vi "gantry移動定位_六邊形(外切圓).vi"() -> ()   [LabVIEW 2016]
uses:
  Classes/Controller/Motion/A3200 Folder/A3200.lvclass
panel:
  out "點座標":dbl[][](array[numeric])
  in  "外切圓半徑":dbl=100.0
  in  "中心點座標":dbl[](array[numeric])
  out "Final Position":dbl[](array[numeric])
  out "Initial position":dbl[](array[numeric])
  in  "Speed (mm/s)":dbl=40.0
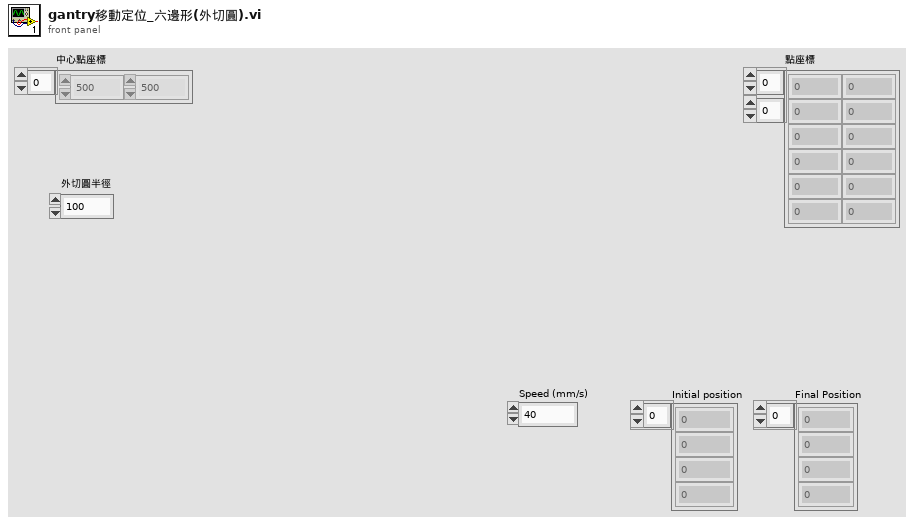
[diagram p1: front panel]
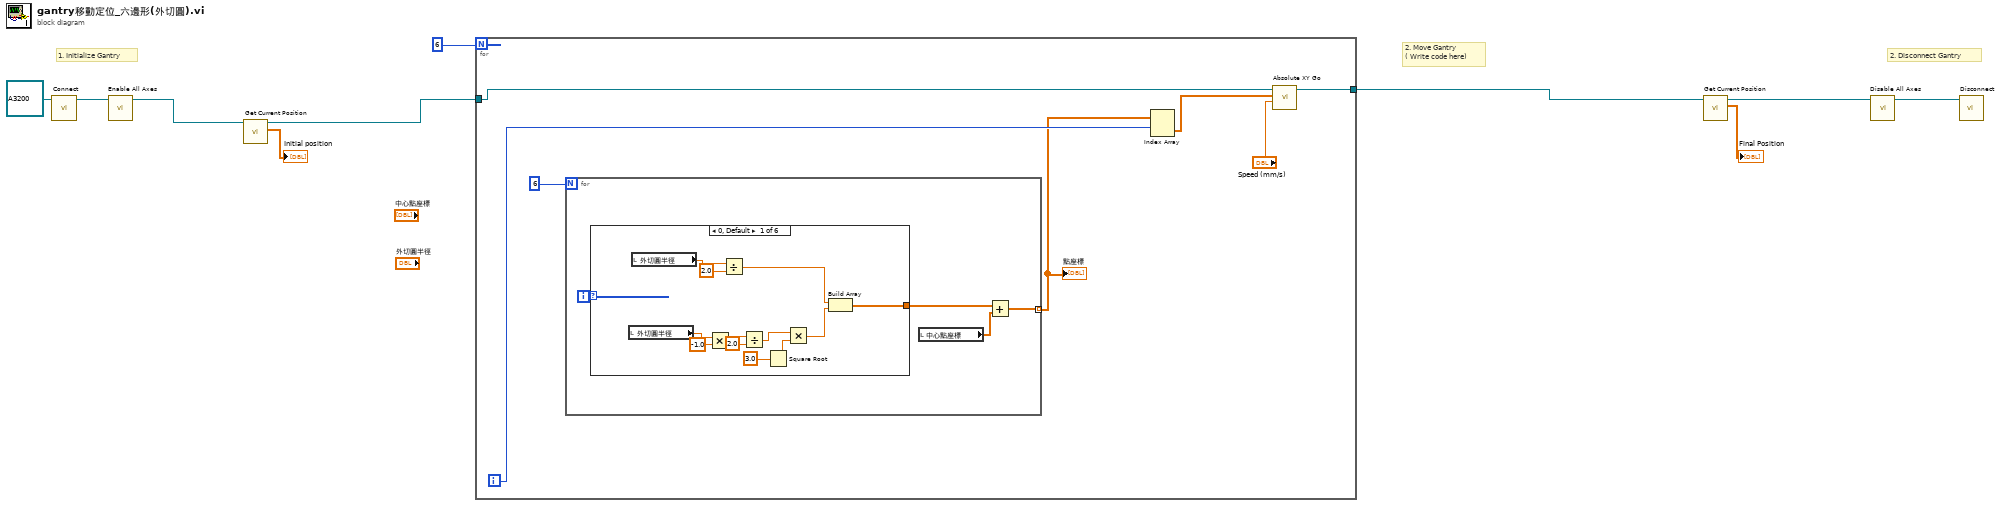
[diagram p0: block diagram]
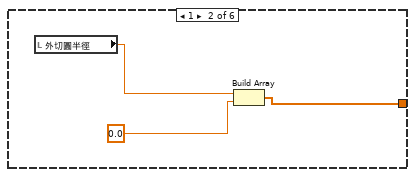
[diagram p2: hidden frame]
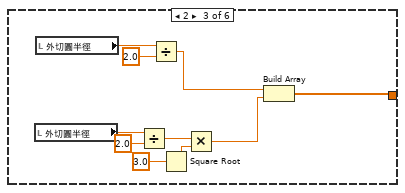
[diagram p3: hidden frame]
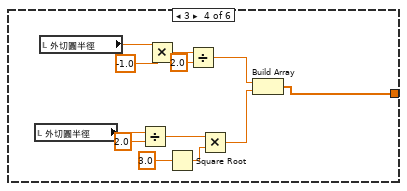
[diagram p4: hidden frame]
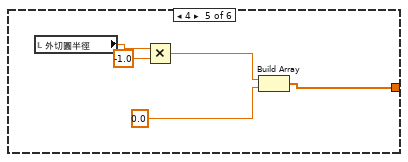
[diagram p5: hidden frame]
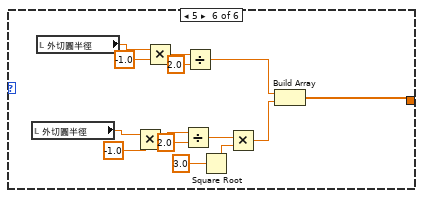
[diagram p6: hidden frame]
diagram:
  # "1. Initialize Gantry"
  # "2. Disconnect Gantry"
  # "2. Move Gantry \n( Write code here)"
  n1 = call-dynamic "Connect.vi"("Gantry in"=refnum<class "A3200.lvclass"> refnum ("A3200.lvclass")) -> ("Gantry out"=w5:refnum<class "A3200.lvclass">)  [unwired: 9 in, 1 out]
  n2 = call-dynamic "Enable All Axes.vi"("A3200 in"=w5) -> ("A3200 out"=w4:refnum<class "A3200.lvclass">)  [unwired: 9 in, 1 out]
  n3 = call-dynamic "Get Current Position.vi"("Gantry in"=w4) -> ("XYZTheta Out"=→"Initial position":dbl[], "Gantry out"=w3:refnum<class "A3200.lvclass">)  [unwired: 8 in, 1 out]
  n4 = for {
    N: 6 -> [_]
    tunnel: w3 -> [w15]
    tunnel: [w14] -> w2
    i -> [w17]
    n5 = for {
      N: 6 -> [_]
      tunnel: [w18] -> w12 mode=indexing
      i -> [w21]
      n6 = case shown="0, Default" w21 {
        tunnel: [w22 w34 w37 w47 w59 w64] -> w20
        frame 0, Default {
          n7 = local read "外切圓半徑"() -> (w30:dbl)
          n8 = local read "外切圓半徑"() -> (w33:dbl)
          n9 = Multiply(x=w30, y=-1.0) -> (x*y=w28:dbl)
          n10 = Divide(x=w33, y=2.0) -> (x/y=w31:dbl)
          n11 = Divide(x=w28, y=2.0) -> (x/y=w26:dbl)
          n12 = Square Root(x=3.0) -> (sqrt(x)=w25:dbl)
          n13 = Multiply(x=w26, y=w25) -> (x*y=w23:dbl)
          n14 = Build Array(w31, w23) -> (w22:dbl[])
        }
        frame 1 {
          n15 = local read "外切圓半徑"() -> (w36:dbl)
          n16 = Build Array(w36, 0.0) -> (w34:dbl[])
        }
        frame 2 {
          n17 = local read "外切圓半徑"() -> (w43:dbl)
          n18 = local read "外切圓半徑"() -> (w46:dbl)
          n19 = Divide(x=w43, y=2.0) -> (x/y=w41:dbl)
          n20 = Divide(x=w46, y=2.0) -> (x/y=w44:dbl)
          n21 = Square Root(x=3.0) -> (sqrt(x)=w40:dbl)
          n22 = Multiply(x=w41, y=w40) -> (x*y=w38:dbl)
          n23 = Build Array(w44, w38) -> (w37:dbl[])
        }
        frame 3 {
          n24 = local read "外切圓半徑"() -> (w53:dbl)
          n25 = local read "外切圓半徑"() -> (w58:dbl)
          n26 = Divide(x=w53, y=2.0) -> (x/y=w51:dbl)
          n27 = Multiply(x=w58, y=-1.0) -> (x*y=w56:dbl)
          n28 = Square Root(x=3.0) -> (sqrt(x)=w50:dbl)
          n29 = Divide(x=w56, y=2.0) -> (x/y=w54:dbl)
          n30 = Multiply(x=w51, y=w50) -> (x*y=w48:dbl)
          n31 = Build Array(w54, w48) -> (w47:dbl[])
        }
        frame 4 {
          n32 = local read "外切圓半徑"() -> (w63:dbl)
          n33 = Multiply(x=w63, y=-1.0) -> (x*y=w61:dbl)
          n34 = Build Array(w61, 0.0) -> (w59:dbl[])
        }
        frame 5 {
          n35 = local read "外切圓半徑"() -> (w72:dbl)
          n36 = local read "外切圓半徑"() -> (w77:dbl)
          n37 = Multiply(x=w72, y=-1.0) -> (x*y=w70:dbl)
          n38 = Multiply(x=w77, y=-1.0) -> (x*y=w75:dbl)
          n39 = Divide(x=w70, y=2.0) -> (x/y=w68:dbl)
          n40 = Divide(x=w75, y=2.0) -> (x/y=w73:dbl)
          n41 = Square Root(x=3.0) -> (sqrt(x)=w67:dbl)
          n42 = Multiply(x=w68, y=w67) -> (x*y=w65:dbl)
          n43 = Build Array(w73, w65) -> (w64:dbl[])
        }
      }
      n44 = local read "中心點座標"() -> (w19:dbl[])
      n45 = Add(x=w20, y=w19) -> (x+y=w18:dbl[])
    }
    "點座標" <- w12
    n46 = Index Array(array=w12, index (row)=w17) -> (element=w11:dbl[])  [unwired: 1 in]
    n47 = call-dynamic "Absolute XY Go.vi"("Speed"="Speed (mm/s)", "XY"=w11, "Gantry in"=w15) -> ("Gantry out"=w14:refnum<class "A3200.lvclass">)  [unwired: 7 in, 1 out]
  }
  n48 = call-dynamic "Get Current Position.vi"("Gantry in"=w2) -> ("XYZTheta Out"=→"Final Position":dbl[], "Gantry out"=w8:refnum<class "A3200.lvclass">)  [unwired: 8 in, 1 out]
  n49 = call-dynamic "Disable All Axes.vi"("Gantry in"=w8) -> ("Gantry out"=w9:refnum<class "A3200.lvclass">)  [unwired: 9 in, 1 out]
  n50 = call-dynamic "Disconnect.vi"("Gantry in"=w9) -> ()  [unwired: 9 in, 1 out]
